vi "InitTilesetBuffer.vi"(8 "error in (no error)":errorcluster, 10 "path to PNG file":path=path "/home/lvuser/natinst/bin/data/UnifiedTileset.png", 11 "Engine in":refnum<class "Engine.lvclass">) -> (0 "error out":errorcluster, 3 "Engine out":refnum<class "Engine.lvclass">)   [LabVIEW 2019, in "RT_Game.lvlib" / "Engine.lvclass"]
uses:
  Engine.lvclass
  Engine.lvclass/Engine.ctl
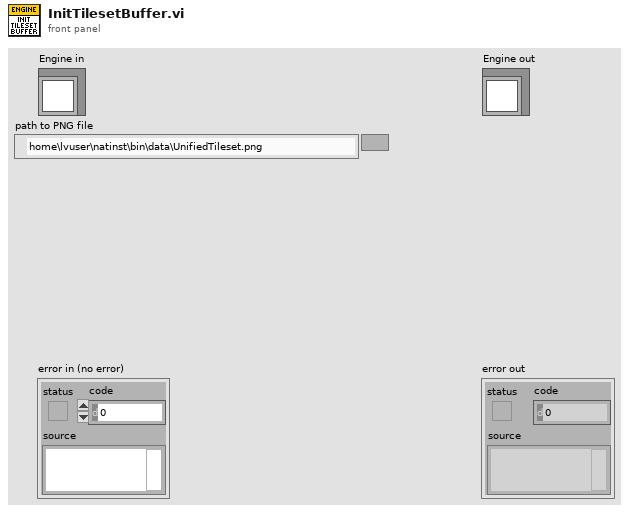
[diagram p1: front panel]
types:
  T1 = typedef "FPGA_Interface.ctl" = refnum<k20>
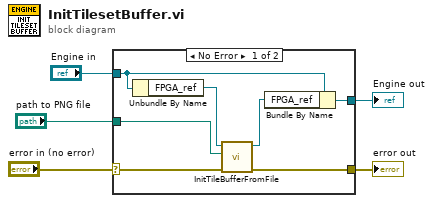
[diagram p0: block diagram]
diagram:
  n1 = case shown="No Error" "error in (no error)" {
    selector: "error in (no error)" -> [w12 w14]
    tunnel: [w9 w14] -> w4
    tunnel: [w10 w13] -> w2
    tunnel: "Engine in" -> [w11 w13]
    tunnel: "path to PNG file" -> [w6 _]
    frame No Error {
      n2 = Unbundle By Name(w11) -> ("FPGA_ref"=w8:T1)
      n3 = call "InitTileBufferFromFile.vi"("error in (no error)"=w12, "Tile Path"=w6, "Refnum in"=w8) -> ("error out"=w9:errorcluster, "Refnum out"=w7:T1)  [unwired: 7 in]
      n4 = Bundle By Name(cluster=w11, "FPGA_ref"=w7) -> (w10:refnum<class "Engine.lvclass">)
    }
    frame Error {
    }
  }
  "error out" <- w4
  "Engine out" <- w2
